vi "Create qlv sheet.vi"() -> ()   [LabVIEW 2019]
uses:
  <vilib>/Utility/file.llb/Read Delimited Spreadsheet (string).vi
  <vilib>/Utility/file.llb/Write Delimited Spreadsheet (string).vi
panel:
  in  "Project":string="1207017361633142"
  out "all rows":string[][](array[string])=[["https://app.asana.com/0/1207017361633142/1207017361633149", "JL1000", "JL1000"], ["https://app.asana.com/0/1207017361633142/1207017361633151", "JL1001", "JL1001"], ["https://app.asana.com/0/1207017361633142/1207017361633153", "JL1002", "JL1002"], ["https://app.asana.com/0/1207017361633142/1207017361633155", "JL1003", "JL1003"], ["https://app.asana.com/0/1207017361633142/1207017361633157", "JL1004", "JL1004"], ["https://app.asana.com/0/1207017361633142/1207017361633159", "JL1005", "JL1005"], ["https://app.asana.com/0/1207017361633142/1207017361633161", "JL1006", "JL1006"], ["https://app.asana.com/0/1207017361633142/1207017361633163", "JL1007", "JL1007"], ["https://app.asana.com/0/1207017361633142/1207017361778778", "JL1008", "JL1008"], ["https://app.asana.com/0/1207017361633142/1207017361778780", "JL1009", "JL1009"], ["https://app.asana.com/0/1207017361633142/1207017361778782", "JL1010", "JL1010"], ["https://app.asana.com/0/1207017361633142/1207017361778784", "JL1011", "JL1011"], ["https://app.asana.com/0/1207017361633142/1207017361778786", "JL1012", "JL1012"], ["https://app.asana.com/0/1207017361633142/1207017361778788", "JL1013", "JL1013"], ["https://app.asana.com/0/1207017361633142/1207017361778790", "JL1014", "JL1014"], ["https://app.asana.com/0/1207017361633142/1207017361778792", "JL1015", "JL1015"], ["https://app.asana.com/0/1207017361633142/1207017361778794", "JL1016", "JL1016"], ["https://app.asana.com/0/1207017361633142/1207017361778796", "JL1017", "JL1017"], ["https://app.asana.com/0/1207017361633142/1207017361778798", "JL1018", "JL1018"], ["https://app.asana.com/0/1207017361633142/1207017361778800", "JL1019", "JL1019"], ["https://app.asana.com/0/1207017361633142/1207017361778802", "JL1020", "JL1020"], ["https://app.asana.com/0/1207017361633142/1207017361778804", "JL1021", "JL1021"], ["https://app.asana.com/0/1207017361633142/1207017361778806", "JL1022", "JL1022"], ["https://app.asana.com/0/1207017361633142/1207017361778808", "JL1023", "JL1023"], ["https://app.asana.com/0/1207017361633142/1207017361778810", "JL1024", "JL1024"], ["https://app.asana.com/0/1207017361633142/1207017361778812", "JL1025", "JL1025"], ["https://app.asana.com/0/1207017361633142/1207017361778814", "JL1026", "JL1026"], ["https://app.asana.com/0/1207017361633142/1207017361778816", "JL1027", "JL1027"], ["https://app.asana.com/0/1207017361633142/1207017361778818", "JL1028", "JL1028"], ["https://app.asana.com/0/1207017361633142/1207017361778820", "JL1029", "JL1029"], ["https://app.asana.com/0/1207017361633142/1207017361778822", "JL1030", "JL1030"], ["https://app.asana.com/0/1207017361633142/1207017361778824", "JL1031", "JL1031"], ["https://app.asana.com/0/1207017361633142/1207017361778826", "JL1032", "JL1032"], ["https://app.asana.com/0/1207017361633142/1207017361778828", "JL1033", "JL1033"], ["https://app.asana.com/0/1207017361633142/1207017361778830", "JL1034", "JL1034"], ["https://app.asana.com/0/1207017361633142/1207017361778832", "JL1035", "JL1035"], ["https://app.asana.com/0/1207017361633142/1207017361778834", "JL1036", "JL1036"], ["https://app.asana.com/0/1207017361633142/1207017361778836", "JL1037", "JL1037"], ["https://app.asana.com/0/1207017361633142/1207017361778838", "JL1038", "JL1038"], ["https://app.asana.com/0/1207017361633142/1207017361778840", "JL1039", "JL1039"], ["https://app.asana.com/0/1207017361633142/1207017361778842", "JL1040", "JL1040"], ["https://app.asana.com/0/1207017361633142/1207017361778844", "JL1041", "JL1041"], ["https://app.asana.com/0/1207017361633142/1207017361778846", "JL1042", "JL1042"], ["https://app.asana.com/0/1207017361633142/1207017361778848", "JL1043", "JL1043"], ["https://app.asana.com/0/1207017361633142/1207017361778850", "JL1044", "JL1044"], ["https://app.asana.com/0/1207017361633142/1207017361778852", "JL1045", "JL1045"], ["https://app.asana.com/0/1207017361633142/1207017361778854", "JL1046", "JL1046"], ["https://app.asana.com/0/1207017361633142/1207017361778856", "JL1047", "JL1047"], ["https://app.asana.com/0/1207017361633142/1207017361778858", "JL1048", "JL1048"], ["https://app.asana.com/0/1207017361633142/1207017361778860", "JL1049", "JL1049"], ["https://app.asana.com/0/1207017361633142/1207017361778862", "JL1050", "JL1050"], ["https://app.asana.com/0/1207017361633142/1207017361778864", "JL1050", "JL1050"], ["https://app.asana.com/0/1207017361633142/1207017361778866", "JL1051", "JL1051"], ["https://app.asana.com/0/1207017361633142/1207017361778868", "JL1052", "JL1052"], ["https://app.asana.com/0/1207017361633142/1207017361778870", "JL1053", "JL1053"], ["https://app.asana.com/0/1207017361633142/1207017361778872", "JL1054", "JL1054"], ["https://app.asana.com/0/1207017361633142/1207017361778874", "JL1055", "JL1055"], ["https://app.asana.com/0/1207017361633142/1207017361778876", "JL1056", "JL1056"], ["https://app.asana.com/0/1207017361633142/1207017361778878", "JL1057", "JL1057"], ["https://app.asana.com/0/1207017361633142/1207017361778880", "JL1058", "JL1058"], ["https://app.asana.com/0/1207017361633142/1207017361778882", "JL1059", "JL1059"], ["https://app.asana.com/0/1207017361633142/1207017361778884", "JL1060", "JL1060"], ["https://app.asana.com/0/1207017361633142/1207017361778886", "JL1061", "JL1061"], ["https://app.asana.com/0/1207017361633142/1207017361778888", "JL1062", "JL1062"], ["https://app.asana.com/0/1207017361633142/1207017361778890", "JL1063", "JL1063"], ["https://app.asana.com/0/1207017361633142/1207017361778892", "JL1064", "JL1064"], ["https://app.asana.com/0/1207017361633142/1207017361778894", "JL1065", "JL1065"], ["https://app.asana.com/0/1207017361633142/1207017361778896", "JL1066", "JL1066"], ["https://app.asana.com/0/1207017361633142/1207017361778898", "JL1067", "JL1067"], ["https://app.asana.com/0/1207017361633142/1207017361778900", "JL1068", "JL1068"], ["https://app.asana.com/0/1207017361633142/1207017361778902", "JL1069", "JL1069"], ["https://app.asana.com/0/1207017361633142/1207017361778904", "JL1070", "JL1070"], ["https://app.asana.com/0/1207017361633142/1207017361778906", "JL1071", "JL1071"], ["https://app.asana.com/0/1207017361633142/1207017361778908", "JL1072", "JL1072"], ["https://app.asana.com/0/1207017361633142/1207017361778910", "JL1073", "JL1073"], ["https://app.asana.com/0/1207017361633142/1207017361778912", "JL1074", "JL1074"], ["https://app.asana.com/0/1207017361633142/1207017361778914", "JL1075", "JL1075"], ["https://app.asana.com/0/1207017361633142/1207017361778916", "JL1076", "JL1076"], ["https://app.asana.com/0/1207017361633142/1207017361778918", "JL1077", "JL1077"], ["https://app.asana.com/0/1207017361633142/1207017361778920", "JL1078", "JL1078"], ["https://app.asana.com/0/1207017361633142/1207017361778922", "JL1079", "JL1079"], ["https://app.asana.com/0/1207017361633142/1207017361778924", "JL1080", "JL1080"], ["https://app.asana.com/0/1207017361633142/1207017361778926", "JL1081", "JL1081"], ["https://app.asana.com/0/1207017361633142/1207017361778928", "JL1082", "JL1082"], ["https://app.asana.com/0/1207017361633142/1207017361778930", "JL1083", "JL1083"], ["https://app.asana.com/0/1207017361633142/1207017361778932", "JL1084", "JL1084"], ["https://app.asana.com/0/1207017361633142/1207017361778934", "JL1085", "JL1085"], ["https://app.asana.com/0/1207017361633142/1207017361778936", "JL1086", "JL1086"], ["https://app.asana.com/0/1207017361633142/1207017361778938", "JL1087", "JL1087"], ["https://app.asana.com/0/1207017361633142/1207017361778940", "JL1088", "JL1088"], ["https://app.asana.com/0/1207017361633142/1207017361778942", "JL1089", "JL1089"], ["https://app.asana.com/0/1207017361633142/1207017361778944", "JL1090", "JL1090"], ["https://app.asana.com/0/1207017361633142/1207017361778946", "JL1091", "JL1091"], ["https://app.asana.com/0/1207017361633142/1207017361778948", "JL1092", "JL1092"], ["https://app.asana.com/0/1207017361633142/1207017361778950", "JL1093", "JL1093"], ["https://app.asana.com/0/1207017361633142/1207017361778952", "JL1094", "JL1094"], ["https://app.asana.com/0/1207017361633142/1207017361778954", "JL1095", "JL1095"], ["https://app.asana.com/0/1207017361633142/1207017361778956", "JL1096", "JL1096"], ["https://app.asana.com/0/1207017361633142/1207017361778958", "JL1097", "JL1097"], ["https://app.asana.com/0/1207017361633142/1207017361778960", "JL1098", "JL1098"], ["https://app.asana.com/0/1207017361633142/1207017361778962", "JL1099", "JL1099"], ["https://app.asana.com/0/1207017361633142/1207017361778964", "JL1100", "JL1100"], ["https://app.asana.com/0/1207017361633142/1207017361778966", "JL1101", "JL1101"], ["https://app.asana.com/0/1207017361633142/1207017361778968", "JL1102", "JL1102"], ["https://app.asana.com/0/1207017361633142/1207017361778970", "JL1103", "JL1103"], ["https://app.asana.com/0/1207017361633142/1207017361778972", "JL1104", "JL1104"], ["https://app.asana.com/0/1207017361633142/1207017361778974", "JL1105", "JL1105"], ["https://app.asana.com/0/1207017361633142/1207017361778976", "JL1106", "JL1106"], ["https://app.asana.com/0/1207017361633142/1207017361778978", "JL1107", "JL1107"], ["https://app.asana.com/0/1207017361633142/1207017361778980", "JL1108", "JL1108"], ["https://app.asana.com/0/1207017361633142/1207017361778982", "JL1109", "JL1109"], ["https://app.asana.com/0/1207017361633142/1207017361778984", "JL1110", "JL1110"], ["https://app.asana.com/0/1207017361633142/1207017361778986", "JL1111", "JL1111"], ["https://app.asana.com/0/1207017361633142/1207017361778988", "JL1112", "JL1112"], ["https://app.asana.com/0/1207017361633142/1207017361778990", "JL1113", "JL1113"], ["https://app.asana.com/0/1207017361633142/1207017361778992", "JL1114", "JL1114"], ["https://app.asana.com/0/1207017361633142/1207017361778994", "JL1115", "JL1115"], ["https://app.asana.com/0/1207017361633142/1207017361778996", "JL1116", "JL1116"], ["https://app.asana.com/0/1207017361633142/1207017361778998", "JL1117", "JL1117"], ["https://app.asana.com/0/1207017361633142/1207017361779000", "JL1118", "JL1118"], ["https://app.asana.com/0/1207017361633142/1207017361779002", "JL1119", "JL1119"], ["https://app.asana.com/0/1207017361633142/1207017361779004", "JL1120", "JL1120"], ["https://app.asana.com/0/1207017361633142/1207017361779006", "JL1121", "JL1121"], ["https://app.asana.com/0/1207017361633142/1207017361779008", "JL1122", "JL1122"], ["https://app.asana.com/0/1207017361633142/1207017361779010", "JL1123", "JL1123"], ["https://app.asana.com/0/1207017361633142/1207017361779012", "JL1124", "JL1124"], ["https://app.asana.com/0/1207017361633142/1207017361779014", "JL1125", "JL1125"], ["https://app.asana.com/0/1207017361633142/1207017361779016", "JL1126", "JL1126"], ["https://app.asana.com/0/1207017361633142/1207017361779018", "JL1127", "JL1127"], ["https://app.asana.com/0/1207017361633142/1207017361779020", "JL1128", "JL1128"], ["https://app.asana.com/0/1207017361633142/1207017361779022", "JL1129", "JL1129"], ["https://app.asana.com/0/1207017361633142/1207017361779024", "JL1130", "JL1130"], ["https://app.asana.com/0/1207017361633142/1207017361779026", "JL1131", "JL1131"], ["https://app.asana.com/0/1207017361633142/1207017361779028", "JL1132", "JL1132"], ["https://app.asana.com/0/1207017361633142/1207017361779030", "JL1133", "JL1133"], ["https://app.asana.com/0/1207017361633142/1207017361779032", "JL1134", "JL1134"], ["https://app.asana.com/0/1207017361633142/1207017361779034", "JL1135", "JL1135"], ["https://app.asana.com/0/1207017361633142/1207017361779036", "JL1136", "JL1136"], ["https://app.asana.com/0/1207017361633142/1207017361779038", "JL1137", "JL1137"], ["https://app.asana.com/0/1207017361633142/1207017361779040", "JL1138", "JL1138"], ["https://app.asana.com/0/1207017361633142/1207017361779042", "JL1139", "JL1139"], ["https://app.asana.com/0/1207017361633142/1207017361779044", "JL1140", "JL1140"], ["https://app.asana.com/0/1207017361633142/1207017361779046", "JL1141", "JL1141"], ["https://app.asana.com/0/1207017361633142/1207017361779048", "JL1142", "JL1142"], ["https://app.asana.com/0/1207017361633142/1207017361779050", "JL1143", "JL1143"], ["https://app.asana.com/0/1207017361633142/1207017361779052", "JL1144", "JL1144"], ["https://app.asana.com/0/1207017361633142/1207017361779054", "JL1145", "JL1145"], ["https://app.asana.com/0/1207017361633142/1207017361779056", "JL1146", "JL1146"], ["https://app.asana.com/0/1207017361633142/1207017361779058", "JL1147", "JL1147"], ["https://app.asana.com/0/1207017361633142/1207017361779060", "JL1148", "JL1148"], ["https://app.asana.com/0/1207017361633142/1207017361779062", "JL1149", "JL1149"], ["https://app.asana.com/0/1207017361633142/1207017361779064", "JL1150", "JL1150"], ["https://app.asana.com/0/1207017361633142/1207017361779066", "JL1151", "JL1151"], ["https://app.asana.com/0/1207017361633142/1207017361779068", "JL1152", "JL1152"], ["https://app.asana.com/0/1207017361633142/1207017361779070", "JL1153", "JL1153"], ["https://app.asana.com/0/1207017361633142/1207017361779072", "JL1154", "JL1154"], ["https://app.asana.com/0/1207017361633142/1207017361779074", "JL1155", "JL1155"], ["https://app.asana.com/0/1207017361633142/1207017361779076", "JL1156", "JL1156"], ["https://app.asana.com/0/1207017361633142/1207017361779078", "JL1157", "JL1157"], ["https://app.asana.com/0/1207017361633142/1207017361779080", "JL1158", "JL1158"], ["https://app.asana.com/0/1207017361633142/1207017361779082", "JL1159", "JL1159"], ["https://app.asana.com/0/1207017361633142/1207017361779084", "JL1160", "JL1160"], ["https://app.asana.com/0/1207017361633142/1207017361779086", "JL1161", "JL1161"], ["https://app.asana.com/0/1207017361633142/1207017361779088", "JL1162", "JL1162"], ["https://app.asana.com/0/1207017361633142/1207017361779090", "JL1163", "JL1163"], ["https://app.asana.com/0/1207017361633142/1207017361779092", "JL1164", "JL1164"], ["https://app.asana.com/0/1207017361633142/1207017361779094", "JL1165", "JL1165"], ["https://app.asana.com/0/1207017361633142/1207017361779096", "JL1166", "JL1166"], ["https://app.asana.com/0/1207017361633142/1207017361779098", "JL1167", "JL1167"], ["https://app.asana.com/0/1207017361633142/1207017361779100", "JL1168", "JL1168"], ["https://app.asana.com/0/1207017361633142/1207017361779102", "JL1169", "JL1169"], ["https://app.asana.com/0/1207017361633142/1207017361779104", "JL1170", "JL1170"], ["https://app.asana.com/0/1207017361633142/1207017361779106", "JL1171", "JL1171"], ["https://app.asana.com/0/1207017361633142/1207017361779108", "JL1172", "JL1172"], ["https://app.asana.com/0/1207017361633142/1207017361779110", "JL1173", "JL1173"], ["https://app.asana.com/0/1207017361633142/1207017361779112", "JL1174", "JL1174"], ["https://app.asana.com/0/1207017361633142/1207017361779114", "JL1175", "JL1175"], ["https://app.asana.com/0/1207017361633142/1207017361779116", "JL1176", "JL1176"], ["https://app.asana.com/0/1207017361633142/1207017361779118", "JL1177", "JL1177"], ["https://app.asana.com/0/1207017361633142/1207017361779120", "JL1178", "JL1178"], ["https://app.asana.com/0/1207017361633142/1207017361779122", "JL1179", "JL1179"], ["https://app.asana.com/0/1207017361633142/1207017361779124", "JL1180", "JL1180"], ["https://app.asana.com/0/1207017361633142/1207017361779126", "JL1181", "JL1181"], ["https://app.asana.com/0/1207017361633142/1207017361779128", "JL1182", "JL1182"], ["https://app.asana.com/0/1207017361633142/1207017361779130", "JL1183", "JL1183"], ["https://app.asana.com/0/1207017361633142/1207017361779132", "JL1184", "JL1184"], ["https://app.asana.com/0/1207017361633142/1207017361779134", "JL1185", "JL1185"], ["https://app.asana.com/0/1207017361633142/1207017361779136", "JL1186", "JL1186"], ["https://app.asana.com/0/1207017361633142/1207017361779138", "JL1187", "JL1187"], ["https://app.asana.com/0/1207017361633142/1207017361779140", "JL1188", "JL1188"], ["https://app.asana.com/0/1207017361633142/1207017361779142", "JL1189", "JL1189"], ["https://app.asana.com/0/1207017361633142/1207017361779144", "JL1190", "JL1190"], ["https://app.asana.com/0/1207017361633142/1207017361779146", "JL1191", "JL1191"], ["https://app.asana.com/0/1207017361633142/1207017361779148", "JL1192", "JL1192"], ["https://app.asana.com/0/1207017361633142/1207017361779150", "JL1193", "JL1193"], ["https://app.asana.com/0/1207017361633142/1207017361779152", "JL1194", "JL1194"], ["https://app.asana.com/0/1207017361633142/1207017361779154", "JL1195", "JL1195"], ["https://app.asana.com/0/1207017361633142/1207017361779156", "JL1196", "JL1196"], ["https://app.asana.com/0/1207017361633142/1207017361779158", "JL1197", "JL1197"], ["https://app.asana.com/0/1207017361633142/1207017361779160", "JL1198", "JL1198"], ["https://app.asana.com/0/1207017361633142/1207017361779162", "JL1199", "JL1199"]]
  in  "file path (dialog if empty)":path
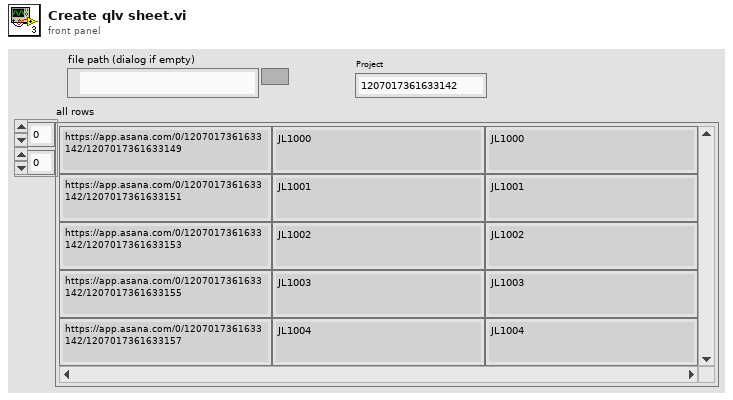
[diagram p1: front panel]
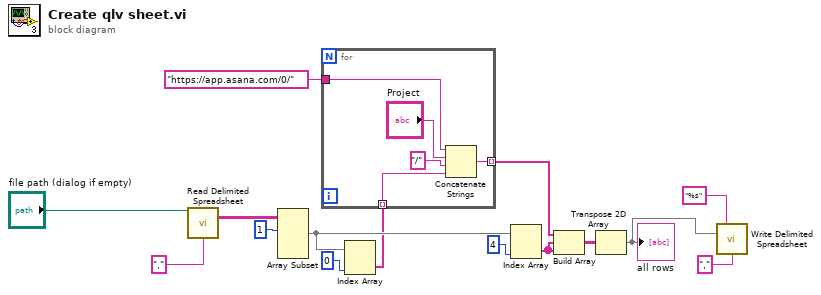
[diagram p0: block diagram]
diagram:
  n1 = call-poly <vilib>:"Read Delimited Spreadsheet.vi"("file path (dialog if empty)"="file path (dialog if empty)", "delimiter (\\t)"="," ("delimiter (\\t)")) -> ("all rows"=w13:string[][])  [unwired: 8 in, 5 out]
  n2 = Array Subset(array=w13, index (row)=1 ("index")) -> (w7:string[][])  [unwired: 3 in]
  n3 = Index Array(array=w7, index (col)=0 ("disabled index (col)")) -> (element=w4:string[])  [unwired: 1 in]
  n4 = for {
    tunnel: [w18] -> w8 mode=indexing
    tunnel: "https://app.asana.com/0/" ("string") -> [w17]
    tunnel: w4 -> [w16] mode=indexing
    n5 = Concatenate Strings(w17, "Project", "/" ("string"), w16) -> (w18:string)
  }
  n6 = Index Array(array=w7, index (col)=4 ("disabled index (col)")) -> (element=w9:string[])  [unwired: 1 in]
  n7 = Build Array(w8, w9, w9) -> (w6:string[][])
  n8 = Transpose 2D Array(2D array=w6) -> (transposed array=w1:string[][])
  "all rows" <- w1
  n9 = call-poly <vilib>:"Write Delimited Spreadsheet.vi"("format (%s)"="%s" ("format (%.3f)"), "2D data"=w1, "delimiter (\\t)"="," ("delimiter (\\t)")) -> ()  [unwired: 11 in, 2 out]
